vi "Frame.Build.Raw.vi"(9 "Fill Byte":u8=255, 10 "Data":u8[](array[numeric])=[0, 0, 0, 0, 0, 0, 0, 0], 11 "identifier":u32) -> (3 "Raw Frame":u8[](array[numeric]))   [LabVIEW 2019, in "Diagnostics Addon Engine.lvlib"]
uses:
  Diagnostics Addon Engine.lvlib
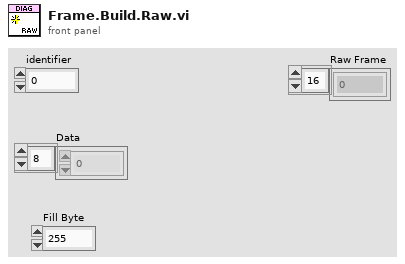
[diagram p1: front panel]
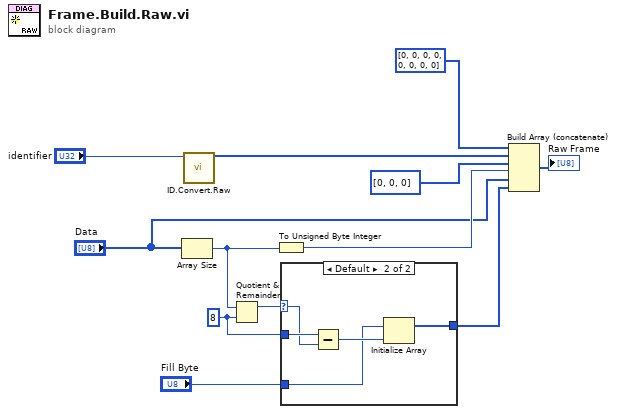
[diagram p0: block diagram]
diagram:
  w4 = 8 ("y")
  n1 = Array Size(array="Data") -> (size(s)=w5:i32)
  n2 = call "ID.Convert.Raw.vi"("identifier"="identifier") -> ("Data"=w11:u8[])  [unwired: 10 in]
  n3 = Quotient & Remainder(x=w5, y=w4) -> (x-y*floor(x/y)=w2:i32)  [unwired: 1 out]
  n4 = To Unsigned Byte Integer(number=w5) -> (unsigned 8bit integer=w8:u8)
  n5 = case shown="Default" w2 {
    selector: w2 -> [_ w14]
    tunnel: w4 -> [_ w17]
    tunnel: [_ w15] -> w3
    tunnel: "Fill Byte" -> [_ w13]
    frame 0 {
    }
    frame Default {
      n6 = Subtract(x=w17, y=w14) -> (x-y=w16:i32)
      n7 = Initialize Array(w13, w16) -> (w15:u8[])
    }
  }
  n8 = Build Array (concatenate)(u8[] [0, 0, 0, 0, 0, 0, 0, 0], w11, u8[] [0, 0, 0], w8, "Data", w3) -> (→"Raw Frame":u8[])
